vi "Read States.vi"(8 "error in (no error)":errorcluster, 11 "HaltTactic in":refnum<class "HaltTactic.lvclass">) -> (0 "error out":errorcluster, 2 "States":enum16{"Halt", "Exit"}(ring), 3 "HaltTactic out":refnum<class "HaltTactic.lvclass">)   [LabVIEW 2023, in "HaltTactic.lvclass"]
uses:
  HaltTactic.lvclass
  HaltTactic.lvclass/HaltTactic.ctl
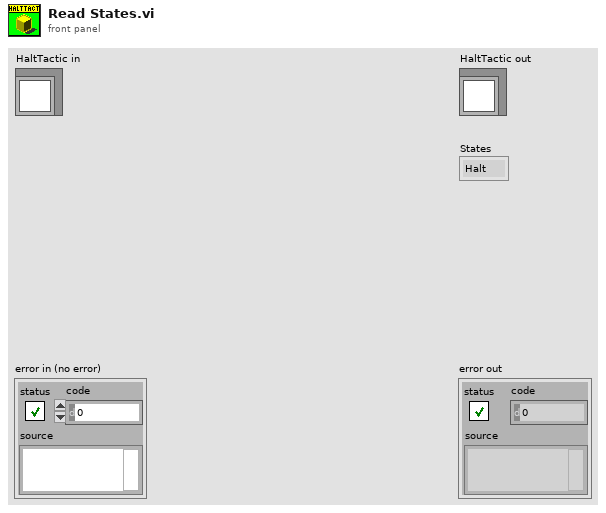
[diagram p1: front panel]
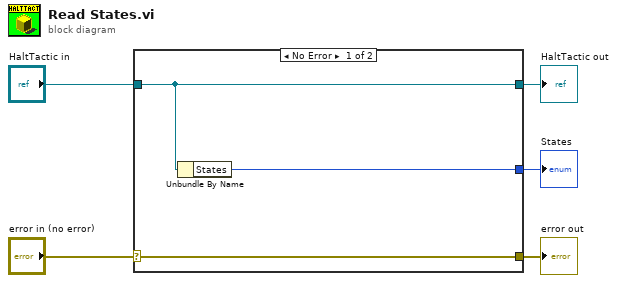
[diagram p0: block diagram]
diagram:
  n1 = case shown="No Error" "error in (no error)" {
    selector: "error in (no error)" -> [w8 w9]
    tunnel: [w8 w9] -> w4
    tunnel: [w7 w10] -> w2
    tunnel: "HaltTactic in" -> [w7 w10]
    tunnel: [w6 _] -> w1
    frame No Error {
      n2 = Unbundle By Name(w7) -> ("States"=w6:enum16{"Halt", "Exit"})
    }
    frame Error {
    }
  }
  "error out" <- w4
  "HaltTactic out" <- w2
  "States" <- w1
